vi "save.vi"(8 "error in (no error)":errorcluster, 10 "Path":path, 11 "DataPointScript in":refnum<class "DataPointScript.lvclass">) -> (0 "error out":errorcluster, 3 "DataPointScript out":refnum<class "DataPointScript.lvclass">)   [LabVIEW 2011, in "Tools.lvlib" / "Scripting.lvlib" / "DataPointScript.lvclass"]
uses:
  DataPointScript.lvclass
  XmlParser.lvclass
  xmlNode/xmlNode.lvclass
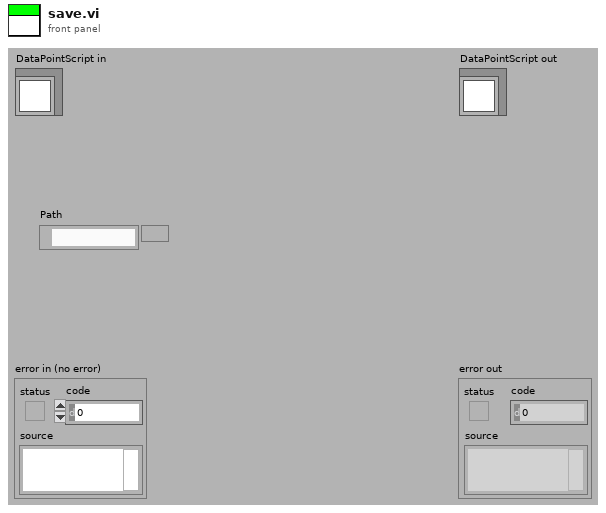
[diagram p1: front panel]
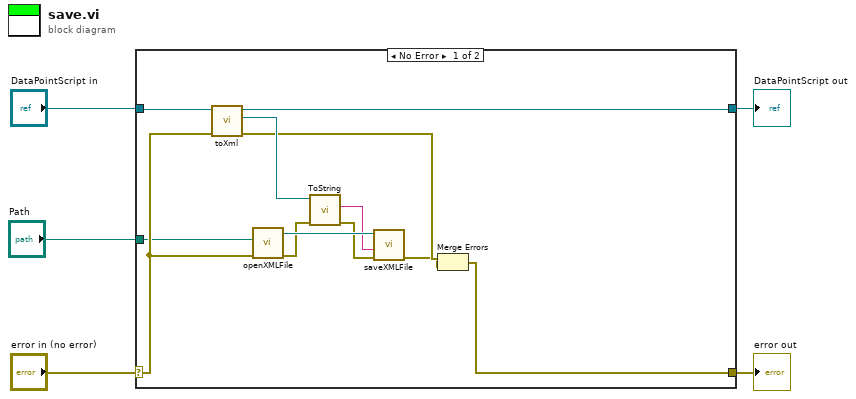
[diagram p0: block diagram]
diagram:
  n1 = case shown="No Error" "error in (no error)" {
    selector: "error in (no error)" -> [w10 w19]
    tunnel: [w6 w19] -> w4
    tunnel: [w16 w18] -> w2
    tunnel: "DataPointScript in" -> [w17 w18]
    tunnel: "Path" -> [w9 _]
    frame No Error {
      n2 = call "toXml.vi"("error in (no error)"=w10, "DataPointScript in"=w17) -> ("error out"=w8:errorcluster, "dataPointXml"=w11:refnum<class "xmlNode.lvclass">, "DataPointScript out"=w16:refnum<class "DataPointScript.lvclass">)  [unwired: 7 in]
      n3 = call "openXMLFile.vi"("error in (no error)"=w10, "Path"=w9) -> ("error out"=w14:errorcluster, "XmlParser out"=w15:refnum<class "XmlParser.lvclass">)  [unwired: 7 in, 1 out]
      n4 = call-dynamic "ToString.vi"("error in (no error)"=w14, "xmlNode in"=w11) -> ("error out"=w13:errorcluster, "xml"=w12:string)  [unwired: 7 in, 1 out]
      n5 = call-dynamic "saveXMLFile.vi"("error in (no error)"=w13, "xmlString"=w12, "XmlParser in"=w15) -> ("error out"=w7:errorcluster)  [unwired: 7 in, 1 out]
      n6 = Merge Errors(w8, w7) -> (w6:errorcluster)
    }
    frame Error {
    }
  }
  "error out" <- w4
  "DataPointScript out" <- w2
